vi "oax_Read Tacho and Vibration Data (Analog Tacho).vi"(7 "reset? (T)":bool=TRUE, 8 "error in (no error)":errorcluster, 11 "refnum":refnum<file>) -> (0 "error out":errorcluster, 1 "channel info":T2[](array[typedef]) {"pregain" format="%.2f"; "weighting filter" items=["Linear", "A-weighting", "B-weighting", "C-weighting", "ITU-R 468-4", "Dolby", "CCITT", "C-message", "Wb", "Wc", "Wd", "We", "Wf", "Wh", "Wj", "Wk", "Wm", "AES17 20 kHz lowpass", "AES17 40 kHz lowpass", "AES17 20 kHz highpass", "AES17 40 kHz highpass"]; "dB reference" format="%^.1e"; "engineering units" items=["custom..."=0, "V"=1, "A"=21, "C"=30, "pC"=31, "s"=32, "-"=29, "Pa"=2, "N"=20, "g"=3, "m/s^2"=4, "m/s"=5, "m"=6, "mm/s"=12, "mm"=13, "micron/s"=14, "micron"=15, "in/s^2"=7, "in/s"=8, "in"=9, "mil/s"=10, "mil"=11, "rad/s^2"=16, "rad/s"=17, "rad"=18, "deg/s^2"=26, "deg/s"=27, "deg"=28, "RPM"=22, "cycle/s^2"=23, "Hz"=24, "cycle"=25, "strain"=19]; "sensor sensitivity" format="%#_5f"}, 2 "waveform data":waveform(dbl)[](array[waveform]), 3 "refnum out":refnum<file>, 4 "channel name":string[](array[string]), 5 "tacho info":T1 {"slope (Rising)" items=["Rising", "Falling"]})   [LabVIEW 2017]
uses:
  <vilib>/addons/_NISVFA/_Shared subVIs/Controls/svc_Channel Info.ctl
  <vilib>/addons/_NISVFA/_Shared subVIs/Controls/svc_Engineering Units Text Ring.ctl
  <vilib>/addons/_NISVFA/_Shared subVIs/Controls/svc_Weighting Filter Text Ring.ctl
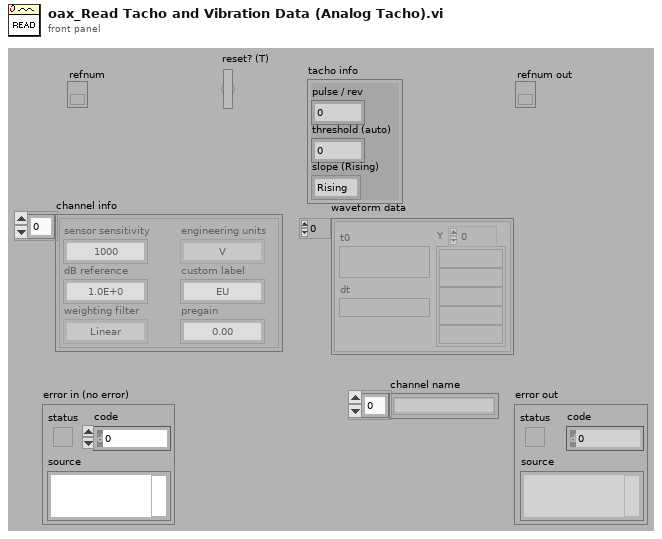
[diagram p1: front panel]
types:
  T1 = cluster{"pulse / rev":i32, "threshold (auto)":dbl, "slope (Rising)":u16}
  T2 = typedef "svc_Channel Info.ctl" = cluster{"sensor sensitivity":dbl, "engineering units":T3, "dB reference":dbl, "custom label":string, "weighting filter":T4, "pregain":dbl}
  T3 = typedef "svc_Engineering Units Text Ring.ctl" = u16
  T4 = typedef "svc_Weighting Filter Text Ring.ctl" = u16
  T5 = cluster{"tacho pulse/rev":i32, "threshold (auto)":dbl, "slope (Rising)":u16}
  T6 = cluster{"pulse / rev":i32, "threshold (auto)":dbl, "slope (Rise)":enum16{"Rise", "Fall"}}
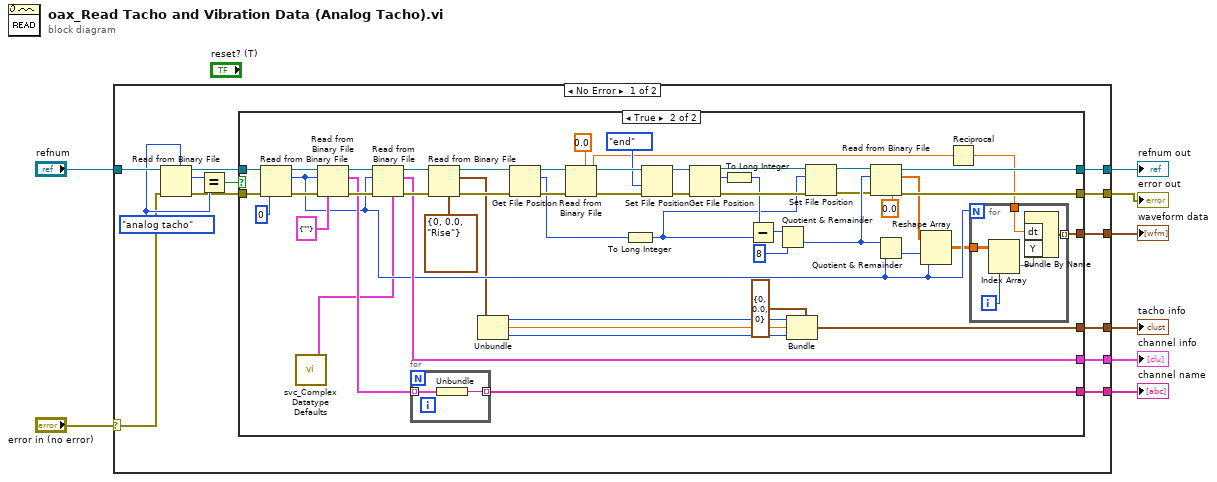
[diagram p0: block diagram]
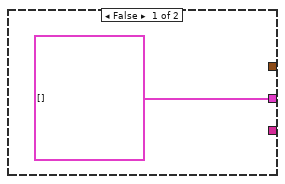
[diagram p2: hidden frame]
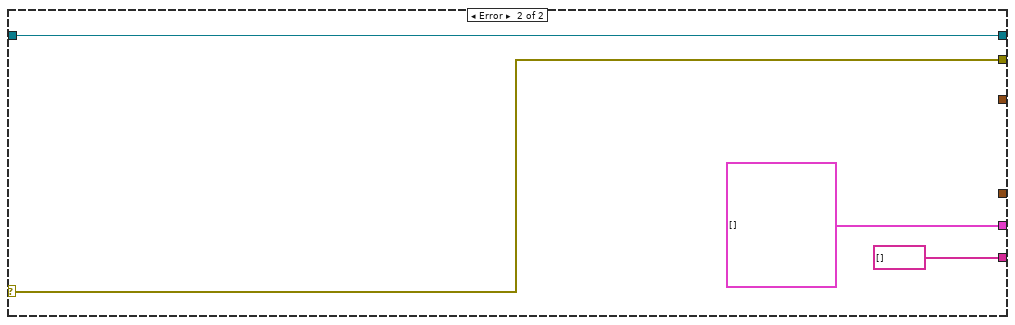
[diagram p3: hidden frame]
diagram:
  n1 = case shown="No Error" "error in (no error)" {
    selector: "error in (no error)" -> [w17 w85]
    tunnel: [w12 w85] -> w7
    tunnel: "refnum" -> [w21 w84]
    tunnel: [w14 w84] -> w4
    tunnel: [w13 _] -> w5
    tunnel: [w11 T2[] []] -> w3
    tunnel: [w10 string[] []] -> w2
    tunnel: [w9 _] -> w1
    frame No Error {
      w19 = enum16{"analog tacho", "digital tacho"}."analog tacho"
      n2 = Read from Binary File(5:w19, 8:w17, 11:w21) -> (0:w15:errorcluster, 2:w20:enum16{"analog tacho", "digital tacho"}, 3:w16:refnum<file>)  [unwired: 3 in, 1 out]
      n3 = Equal?(x=w20, y=w19) -> (x = y?=w18:bool)
      n4 = case shown="True" w18 {
        tunnel: w16 -> [_ w73]
        tunnel: w15 -> [_ w74]
        tunnel: [_ w57] -> w14
        tunnel: [_ w23] -> w13
        tunnel: [_ w58] -> w12
        tunnel: [T2[] [] w66] -> w11
        tunnel: [_ w59] -> w10
        tunnel: [_ w45] -> w9
        frame False {
        }
        frame True {
          n5 = Read from Binary File(5:0, 8:w74, 11:w73) -> (0:w65:errorcluster, 2:w39:i32, 3:w63:refnum<file>)  [unwired: 3 in, 1 out]
          n6 = call <vilib>:"svc_Complex Datatype Defaults.vi"() -> ("channel info"=w29:T2)  [unwired: 11 in, 8 out]
          n7 = Read from Binary File(5:cluster{"ch0 string":string} {"ch0 string"=""}, 8:w65, 10:w39, 11:w63) -> (0:w64:errorcluster, 2:w60:cluster{"ch0 string":string}[], 3:w62:refnum<file>)  [unwired: 2 in, 1 out]
          n8 = Read from Binary File(5:w29, 8:w64, 10:w39, 11:w62) -> (0:w68:errorcluster, 2:w66:T2[], 3:w67:refnum<file>)  [unwired: 2 in, 1 out]
          n9 = for {
            tunnel: w60 -> [w81] mode=indexing
            tunnel: [w80] -> w59 mode=indexing
            n10 = Unbundle(w81) -> ("ch0 string"=w80:string)
          }
          n11 = Read from Binary File(5:T6 {"pulse / rev"=0, "threshold (auto)"=0.0, "slope (Rise)"=enum."Rise"} ("tacho info"), 8:w68, 11:w67) -> (0:w70:errorcluster, 2:w28:T6, 3:w69:refnum<file>)  [unwired: 3 in, 1 out]
          n12 = Unbundle(w28) -> ("pulse / rev"=w26:i32, "threshold (auto)"=w25:dbl, "slope (Rise)"=w24:enum16{"Rise", "Fall"})
          n13 = Read from Binary File(5:0.0 ("1/x"), 8:w70, 11:w69) -> (0:w31:errorcluster, 2:w46:dbl, 3:w32:refnum<file>)  [unwired: 3 in, 1 out]
          n14 = Get File Position(4:w31, 7:w32) -> (0:w54:errorcluster, 2:w30:i64, 3:w55:refnum<file>)
          n15 = To Long Integer(number=w30) -> (32bit integer=w40:i32)
          n16 = Set File Position(refnum=w55, from (0:start)=enum16{"start", "end", "current"}."end" ("pos mode (0:2)"), error in=w54) -> (refnum out=w37:refnum<file>, error out=w36:errorcluster)  [unwired: 1 in]
          n17 = Get File Position(4:w36, 7:w37) -> (0:w53:errorcluster, 2:w35:i64, 3:w52:refnum<file>)
          n18 = To Long Integer(number=w35) -> (32bit integer=w50:i32)
          n19 = Subtract(x=w50, y=w40) -> (x-y=w49:i32)
          n20 = Quotient & Remainder(x=w49, y=8) -> (floor(x/y)=w42:i32)  [unwired: 1 out]
          n21 = Bundle(cluster=T5 {"tacho pulse/rev"=0, "threshold (auto)"=0.0, "slope (Rising)"=0}, "tacho pulse/rev"=w26, "threshold (auto)"=w25, "slope (Rising)"=w24) -> (w23:T5)
          n22 = Set File Position(offset (in bytes) (0)=w40, refnum=w52, error in=w53) -> (refnum out=w34:refnum<file>, error out=w33:errorcluster)  [unwired: 1 in]
          n23 = Read from Binary File(5:0.0 ("1/x"), 8:w33, 10:w42, 11:w34) -> (0:w58:errorcluster, 2:w43:dbl[], 3:w57:refnum<file>)  [unwired: 2 in, 1 out]
          n24 = Quotient & Remainder(x=w42, y=w39) -> (floor(x/y)=w41:i32)  [unwired: 1 out]
          n25 = Reshape Array(w43, w41, w39) -> (w38:dbl[][])
          n26 = Reciprocal(x=w46) -> (1/x=w44:dbl)
          n27 = for {
            N: w39 -> [_]
            tunnel: w44 -> [w79]
            tunnel: [w78] -> w45 mode=indexing
            tunnel: w38 -> [w77]
            i -> [w76]
            n28 = Index Array(array=w77, index (col)=w76) -> (element=w75:dbl[])  [unwired: 1 in]
            n29 = Bundle By Name("dt"=w79, "Y"=w75) -> (w78:waveform(dbl))  [unwired: 1 in]
          }
        }
      }
    }
    frame Error {
    }
  }
  "error out" <- w7
  "channel info" <- w3
  "waveform data" <- w1
  "tacho info" <- w5
  "refnum out" <- w4
  "channel name" <- w2
